vi "RunTest2.vi"(8 "error in (no error)":errorcluster, 11 "Prueba02 in":refnum<class "Prueba02.lvclass">) -> (0 "error out":errorcluster, 2 "resultado":string, 3 "Prueba02 out":refnum<class "Prueba02.lvclass">)   [LabVIEW 2019, in "Prueba02.lvclass"]
uses:
  Prueba02.lvclass
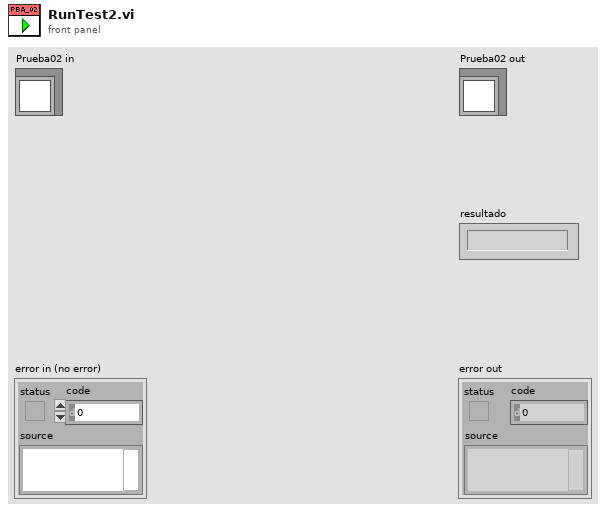
[diagram p1: front panel]
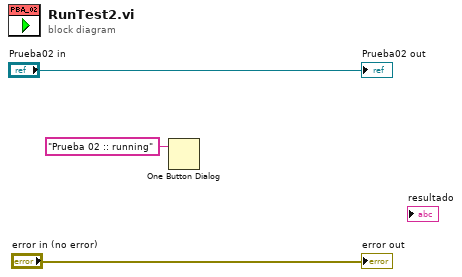
[diagram p0: block diagram]
diagram:
  n1 = One Button Dialog(message="Prueba 02 :: running") -> ()  [unwired: 1 in, 1 out]
  "error out" <- "error in (no error)"
  "Prueba02 out" <- "Prueba02 in"
